vi "Exercise 5-2.vi"() -> ()   [LabVIEW 2014]
panel:
  out "Small Cluster":cluster{"Boolean 1":bool, "Slide":dbl} {"Slide" scale=0.0..10.0}
  out "Modified Cluster":T1 {"Slide" scale=0.0..10.0}
  in  "Cluster":T1 {"Slide" scale=0.0..10.0}
  out "Boolean 2":bool
  out "Numeric":dbl
  in  "stop":bool
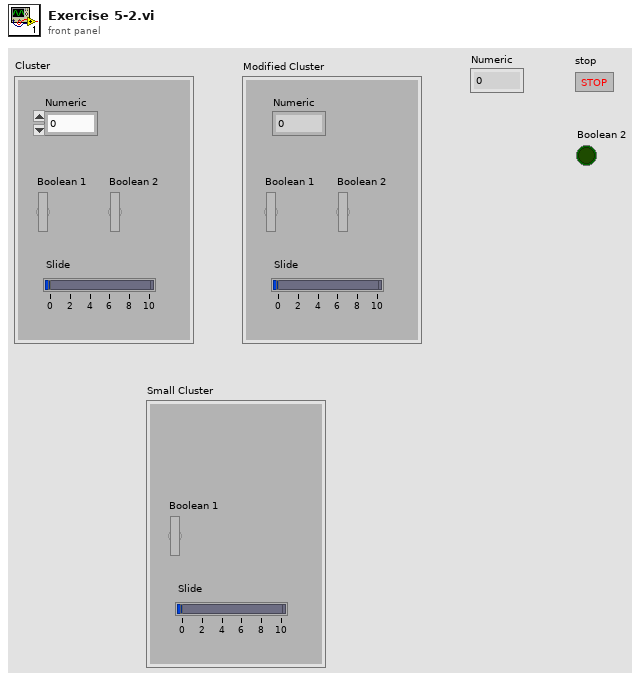
[diagram p1: front panel]
types:
  T1 = cluster{"Numeric":dbl, "Boolean 1":bool, "Boolean 2":bool, "Slide":dbl}
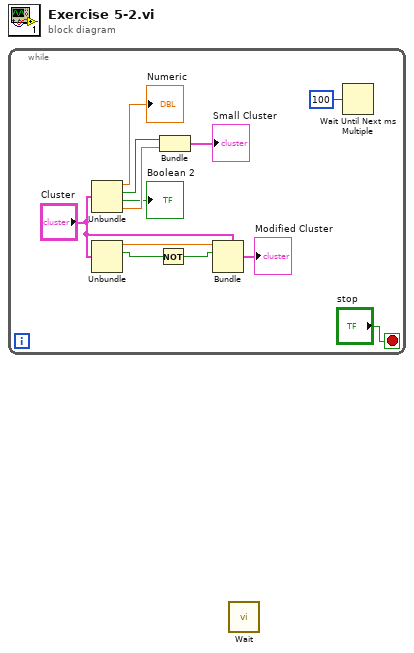
[diagram p0: block diagram]
diagram:
  n1 = while {
    stop <- "stop" stop-if-true
    n2 = Unbundle("Cluster") -> ("Numeric"=→"Numeric":dbl, "Boolean 1"=w11:bool, "Boolean 2"=→"Boolean 2":bool, "Slide"=w10:dbl)
    n3 = Unbundle("Cluster") -> ("Numeric"=w6:dbl, "Boolean 1"=w5:bool)  [unwired: 2 out]
    n4 = Not(x=w5) -> (.not. x?=w4:bool)
    n5 = Bundle("Boolean 1"=w11, "Slide"=w10) -> (→"Small Cluster":cluster{"Boolean 1":bool, "Slide":dbl})  [unwired: 1 in]
    n6 = Bundle(cluster="Cluster", "Numeric"=w6, "Boolean 1"=w4) -> (→"Modified Cluster":T1)  [unwired: 2 in]
    n7 = Wait Until Next ms Multiple(millisecond multiple=u32 100) -> ()  [unwired: 1 out]
  }
  n8 = call "Wait"() -> ()  [unwired: 1 in, 1 out]
